vi "OAT Remove Slow Roll Error (Multi Channels).vi"(6 "phase setting":T1, 7 "reset? (True)":bool=TRUE, 8 "error in (no error)":errorcluster, 9 "slow roll vectors":cdb[][](array[numeric]) format="%.2f", 10 "phase lags":cluster{"X":dbl[], "Y":dbl[]}[][](array[cluster]) {"Y" format="%.2f"; "X" format="%.2f"}, 11 "magnitudes (RMS)":cluster{"X":dbl[], "Y":dbl[]}[][](array[cluster]) {"Y" format="%.2f"; "X" format="%.2f"}) -> (0 "error out":errorcluster, 1 "actual slow roll vectors":cdb[][](array[numeric]) format="%.2f", 2 "compensated phase lags":cluster{"X":dbl[], "Y":dbl[]}[][](array[cluster]) {"Y" format="%.2f"; "X" format="%.2f"}, 3 "compensated magnitudes (RMS)":cluster{"X":dbl[], "Y":dbl[]}[][](array[cluster]) {"Y" format="%.2f"; "X" format="%.2f"})   [LabVIEW 2017]
doc: "Performs run out compensation for proximity probe signals sampled from multiple channels. This vi receives <B>magnitudes (RMS)</B> and <B>phase lags</B> from the order tracking vis and the <B>slow roll vectors</B> of the same orders.It removes the slow roll errors by subtracting the <B>slow roll vectors</B> from the corresponding <B>magnitudes (RMS)</B> and <B>phase lags</B>."
uses:
  <vilib>/addons/Sound and Vibration/Order Analysis/Misc/OAT Convert Phase (N Channels).vi
  <vilib>/Analysis/NI_AALPro.lvlib
  <vilib>/addons/Sound and Vibration/Order Analysis/Resample Order Tracking/SoundVib_Resampling.lvlib
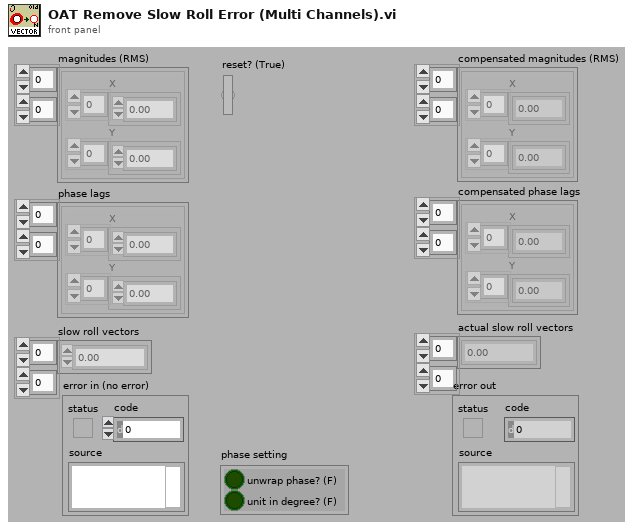
[diagram p1: front panel]
types:
  T1 = cluster{"unwrap phase? (F)":bool, "unit in degree? (F)":bool}
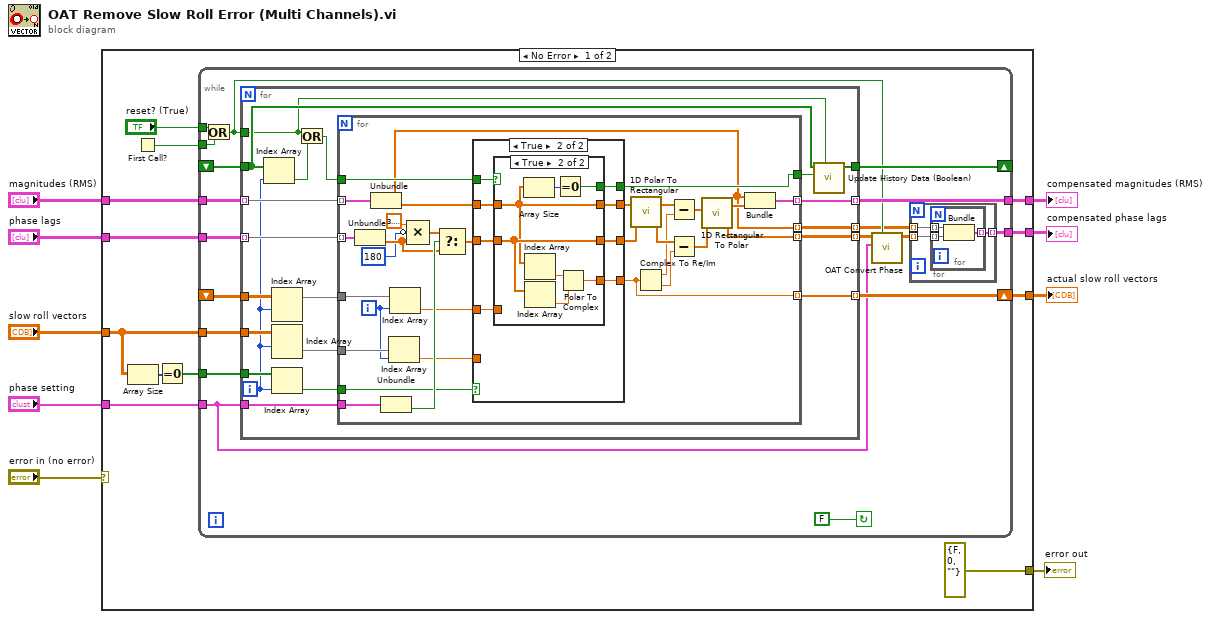
[diagram p0: block diagram]
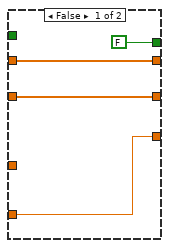
[diagram p2: hidden frame]
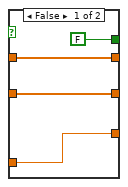
[diagram p3: hidden frame]
diagram:
  n1 = case shown="No Error" "error in (no error)" {
    selector: "error in (no error)" -> [_ w123]
    tunnel: "magnitudes (RMS)" -> [w11 w122]
    tunnel: "phase lags" -> [w21 w121]
    tunnel: "slow roll vectors" -> [w14 w120]
    tunnel: [w20 w122] -> w6
    tunnel: [w10 w121] -> w5
    tunnel: [errorcluster {"status"=FALSE, "code"=0, "source"=""} ("error IO") w123] -> w3
    tunnel: [w18 w120] -> w2
    tunnel: "phase setting" -> [w16 _]
    frame No Error {
      n2 = Array Size(array=w14) -> (size(s)=w17:i32[])
      n3 = First Call?() -> (First Call?: T/F=w13:bool)
      n4 = Equal To 0?(x=w17) -> (x = 0?=w15:bool[])
      n5 = while {
        tunnel: w11 -> [w37]
        tunnel: w21 -> [w36]
        tunnel: [w39] -> w20
        shift-right: [w35] -> w18
        shift-left: _ -> [w34]
        tunnel: w16 -> [w28]
        tunnel: w15 -> [w33]
        tunnel: w14 -> [w32]
        shift-right: [w30] -> _
        shift-left: _ -> [w31]
        tunnel: w13 -> [w26]
        tunnel: "reset? (True)" -> [w27]
        tunnel: [w22] -> w10
        stop <- FALSE continue-if-true
        n6 = Or(x=w27, y=w26) -> (x .or. y?=w25:bool)
        n7 = for {
          tunnel: [w65] -> w39 mode=indexing
          tunnel: w37 -> [w64] mode=indexing
          tunnel: w36 -> [w63] mode=indexing
          tunnel: [w62] -> w35 mode=indexing
          tunnel: w34 -> [w60]
          tunnel: w28 -> [w61]
          tunnel: w33 -> [w56]
          tunnel: w32 -> [w58]
          tunnel: w31 -> [w52]
          tunnel: [w53] -> w30
          tunnel: [w48] -> w24 mode=indexing
          tunnel: [w47] -> w29 mode=indexing
          tunnel: w25 -> [w46]
          i -> [w49]
          n8 = Index Array(array=w52, index=w49) -> (element=w51:bool)
          n9 = Index Array(array=w60, index (row)=w49) -> (element=w59:cdb[])  [unwired: 1 in]
          n10 = Index Array(array=w58, index (row)=w49) -> (element=w57:cdb[])  [unwired: 1 in]
          n11 = Index Array(array=w56, index=w49) -> (element=w55:bool)
          n12 = Or(x=w46, y=w51) -> (x .or. y?=w50:bool)
          n13 = for {
            tunnel: w64 -> [w96] mode=indexing
            tunnel: w63 -> [w95] mode=indexing
            tunnel: [w94] -> w65 mode=indexing
            tunnel: [w78] -> w62 mode=indexing
            tunnel: w59 -> [w77]
            tunnel: w50 -> [w93]
            tunnel: w61 -> [w81]
            tunnel: w55 -> [w73]
            tunnel: w57 -> [w75]
            tunnel: [w68] -> w54
            tunnel: [w67] -> w48 mode=indexing
            tunnel: [w66] -> w47 mode=indexing
            i -> [w74]
            n14 = Unbundle(w95) -> ("Y"=w71:dbl[])  [unwired: 1 out]
            n15 = Unbundle(w96) -> ("X"=w67:dbl[], "Y"=w92:dbl[])
            n16 = Unbundle(w81) -> ("unit in degree? (F)"=w84:bool)  [unwired: 1 out]
            n17 = Index Array(array=w75, index=w74) -> (element=w72:cdb)
            n18 = Index Array(array=w77, index=w74) -> (element=w76:cdb)
            n19 = Compound Arithmetic op=MULTIPLY(3.141592653589793, invert 180, w71) -> (w82:dbl[])
            n20 = Select(t=w82, s=w84, f=w71) -> (s? t:f=w83:dbl[])
            n21 = case shown="True" w73 {
              tunnel: w93 -> [_ w108]
              tunnel: w92 -> [w98 w107]
              tunnel: [w98 w106] -> w91
              tunnel: [w99 w105] -> w90
              tunnel: w83 -> [w99 w104]
              tunnel: [w100 w103] -> w78
              tunnel: w76 -> [_ w102]
              tunnel: w72 -> [w100 _]
              tunnel: [FALSE w101] -> w68
              frame False {
              }
              frame True {
                n22 = case shown="True" w108 {
                  tunnel: w107 -> [w111 w115]
                  tunnel: [w112 w116] -> w103
                  tunnel: w104 -> [w110 w119]
                  tunnel: w102 -> [w112 _]
                  tunnel: [w111 w115] -> w106
                  tunnel: [w110 w119] -> w105
                  tunnel: [FALSE w113] -> w101
                  frame False {
                  }
                  frame True {
                    n23 = Array Size(array=w115) -> (size(s)=w114:i32)
                    n24 = Index Array(array=w115) -> (element=w118:dbl)  [unwired: 1 in]
                    n25 = Index Array(array=w119) -> (element=w117:dbl)  [unwired: 1 in]
                    n26 = Equal To 0?(x=w114) -> (x = 0?=w113:bool)
                    n27 = Polar To Complex(1:w117, 2:w118) -> (0:w116:cdb)
                  }
                }
              }
            }
            n28 = call <vilib>:"1D Polar To Rectangular.vi"("Magnitude"=w91, "Phase"=w90) -> ("X"=w89:dbl[], "Y"=w88:dbl[])  [unwired: 1 out]
            n29 = Complex To Re/Im(x + iy=w78) -> (x=w80:dbl, y=w79:dbl)
            n30 = Subtract(x=w89, y=w80) -> (x-y=w87:dbl[])
            n31 = Subtract(x=w88, y=w79) -> (x-y=w86:dbl[])
            n32 = call <vilib>:"1D Rectangular To Polar.vi"("X"=w87, "Y"=w86) -> ("Magnitude"=w85:dbl[], "Phase"=w66:dbl[])  [unwired: 1 out]
            n33 = Bundle("X"=w67, "Magnitude"=w85) -> (w94:cluster{"X":dbl[], "Magnitude":dbl[]})  [unwired: 1 in]
          }
          n34 = call <vilib>:"Update History Data (Boolean).vi"("reset?"=w46, "new data"=w54, "History Data In"=w52) -> ("History Data Out"=w53:bool[])  [unwired: 8 in]
        }
        n35 = call-poly <vilib>:"OAT Convert Phase.vi"("reset (TRUE)"=w25, "desired phase setting"=w28, "phase in"=w29) -> ("phase out"=w23:dbl[][][])  [unwired: 8 in]
        n36 = for {
          tunnel: w24 -> [w42] mode=indexing
          tunnel: w23 -> [w41] mode=indexing
          tunnel: [w40] -> w22 mode=indexing
          n37 = for {
            tunnel: w42 -> [w44] mode=indexing
            tunnel: w41 -> [w45] mode=indexing
            tunnel: [w43] -> w40 mode=indexing
            n38 = Bundle("X"=w44, "phase out"=w45) -> (w43:cluster{"X":dbl[], "phase out":dbl[]})  [unwired: 1 in]
          }
        }
      }
    }
    frame Error {
    }
  }
  "error out" <- w3
  "compensated magnitudes (RMS)" <- w6
  "compensated phase lags" <- w5
  "actual slow roll vectors" <- w2
